vi "oax_gsTacho Analyzer.vi"() -> ()   [LabVIEW 2017]
doc: "<B>Tach Signal Analyzer</B>\n\nUse the Tach Signal Analyzer to prepare data samples for order tracking. The raw data can be input from either a binary NI-DAQ file collected by the <B>DSA Data Logger</B> or a general Windows .wav file. In this demo application, the usable data is limited to the data files come along with it.\n\nBy adjusting the <B>Selected Order</B> control in the <B>Time-Frequency Plot Parameters</B> section of the front panel, you can see a black curve moving around in the <B>Time-Frequency Plot</B>. The black curve represents the instantaneous frequencies of the selected order. You can increase the mask width to make the black curve more visible. For accurate order tracking, the black curve must be right on top of the corresponding orders displayed in the <B>Time-Frequency Plot</B>. You can use the controls in the <B>Tachometer Control</B> section to alter the black curve for a better fit.\n\nIn addition to verifying computed instantaneous frequencies, the <B>Tach Signal Analyzer</B> also allows you to select the most interesting events and to remove unwanted samples from the data record. For the sake of computation speed, it is important to keep the number of analyzed data samples as small as possible.\n\nOnce you have a good fit of the black curve on the corresponding orders in the <B>Time-Frequency Plot</B>, choose <B>File >> Save</B> on the toolbar to create an intermediate data file for order analysis."
uses:
  <vilib>/addons/Sound and Vibration/Order Analysis/Tach Process/SubVIs/speed profile.ctl
  <vilib>/addons/Sound and Vibration/Order Analysis/Ref Gabor Order Tracking/window information.ctl
  <vilib>/Analysis/1siggen.llb/Ramp Pattern by Samples.vi
  <vilib>/addons/Sound and Vibration/Order Analysis/Ref Gabor Order Tracking/Get Freq-Time Spectral Map (U8).vi
  Instance           2 28Saved   oax_gsTacho Analyzer .vi
  Instance           1 28Saved   oax_gsTacho Analyzer .vi
  <vilib>/addons/Sound and Vibration/Order Analysis/Example Support/Demo VI/Start-Up Kit/OAT Start/global variable.vi
  <vilib>/addons/Sound and Vibration/Order Analysis/Tach Process/SoundVib_TachProcess.lvlib
  <vilib>/addons/Sound and Vibration/Order Analysis/Gabor Order Tracking/SoundVib_Gabor.lvlib
  <vilib>/Analysis/NI_AALBase.lvlib
panel:
  in  "Save":bool
  in  "Select Data":string(tree)="UpAcc.wav"
  out "check sum":i16[](array[numeric])
  out "file names":string[](array[string])
  in  "unit":u16(ring) items=["Order", "Hz"]
  in  "Bandwidth":dbl(slide)=0.5 min=0.0 scale=0.0..1.0 scale format="%.2p"
  out "window information":T1={"window type"=3, "window length"=1} {"window type" items=["None"=0, "Hanning"=1, "Hamming"=2, "Blackman-Harris"=3, "Exact Blackman"=4, "Blackman"=5, "Flat Top"=6, "4 Term B-Harris"=7, "7 Term B-Harris"=8, "Low Sidelobe"=9, "Gaussian"=62]; "window length" min=0}
  out "Sample Rate (Hz)":dbl
  out "S&V plot":dbl[](graph)
  in  "Missing\nPulses?":bool
  in  "Threshold":bool
  in  "threshold lvl":dbl
  out "Num. of Data Selected":i32
  out "file start":i32=414
  out "Status":string="Waiting ..."
  out "Pulse Info":T2 {"speed [RPM]" format="%.2f"; "time [s]" format="%.2f"}
  in  "Pulses/Rev":i32=2
  in  "Window Length":T3(ring)=enum."2048"
  in  "Selected Order":dbl=1.0 min=0.1 step=0.1 format="%.1f"
  in  "Slope":enum16{"Rise", "Fall"}(ring)
  in  "Detrend":dbl(slide) min=0.0 max=1.0 step=0.05 scale=0.0..1.0 scale format="%.2f"
  out "Sound or Vibration Data":string
  out "Tachometer Data":string
  out "tach plot":cluster{dbl[], dbl[]}[](graph)
  out "Time-Frequency Plot":u8[][](graph)
  # "Time-Frequency Plot \nParameters"
  # "narrow"
  # "wide"
  # "Tachometer Control"
  # "Save Data"
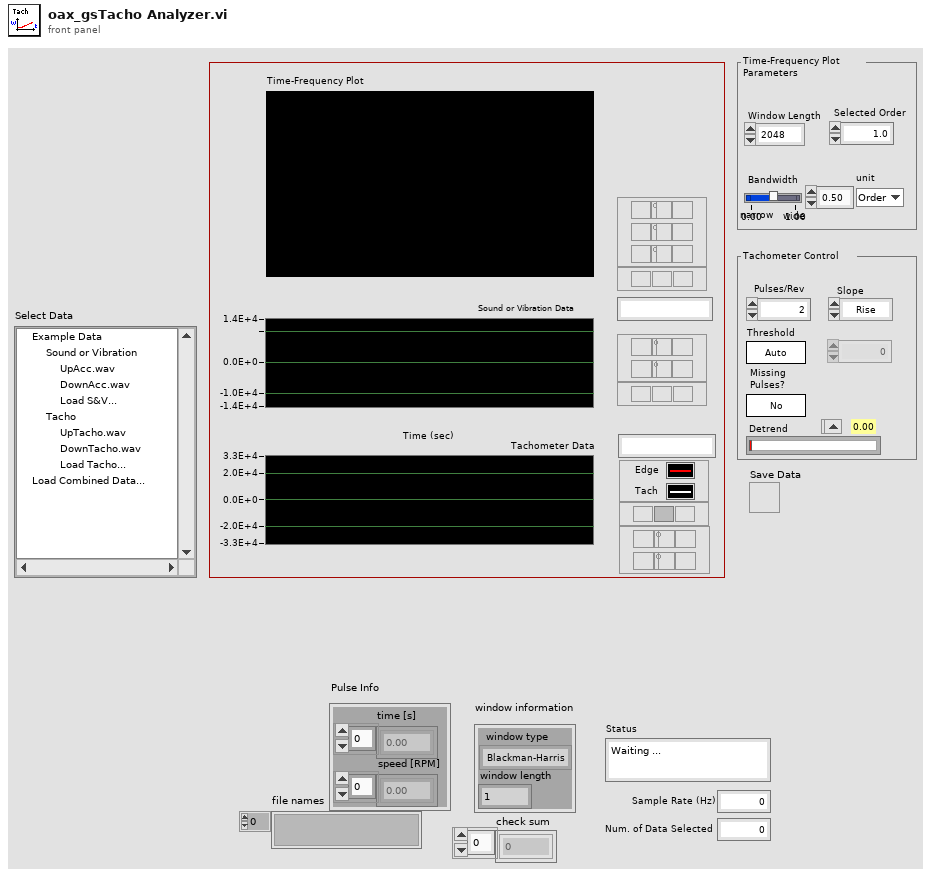
[diagram p1: front panel]
types:
  T1 = typedef "SoundVib_Gabor.lvlib/window information.ctl" = cluster{"window type":u32, "window length":i32}
  T2 = typedef "SoundVib_TachProcess.lvlib/speed profile.ctl" = cluster{"time [s]":dbl[], "speed [RPM]":dbl[]}
  T3 = enum16{"1024", "2048", "4096", "8192", "16384", "32768"}
  T4 = cluster{"Tach processed":bool, "SV processed":bool, "sample rate":u32}
  T5 = cluster{"Bandwidth":dbl, "unit":u16, "Selected Order":dbl}
  T6 = cluster{"Pulses/Rev":i32, "Detrend":dbl, "Slope":enum16{"Rise", "Fall"}, "Missing\nPulses?":bool, "threshold lvl":dbl, "Threshold":bool}
  T7 = typedef "Sound Format+.ctl" = cluster{"quality":enum16{"mono", "stereo"}, "sample rate":u32, "bits/sample":enum16{"8 bit", "16 bit"}}
  T8 = typedef "SoundVib_Gabor.lvlib/GT RefNum.ctl" = refnum<k1>
  T9 = cluster{"name":string, "multiplier":sgl, "offset":sgl, "sensor sensitivity (mV/EU)":dbl, "engineering units":enum16{"custom...", "V", "Pa", "g", "m/s^2", "m/s", "m", "in/s^2", "in/s", "in"}}[]
  T10 = cluster{"YScale.NameLbl.Text":string, "YScale.NameLbl.Text":string}
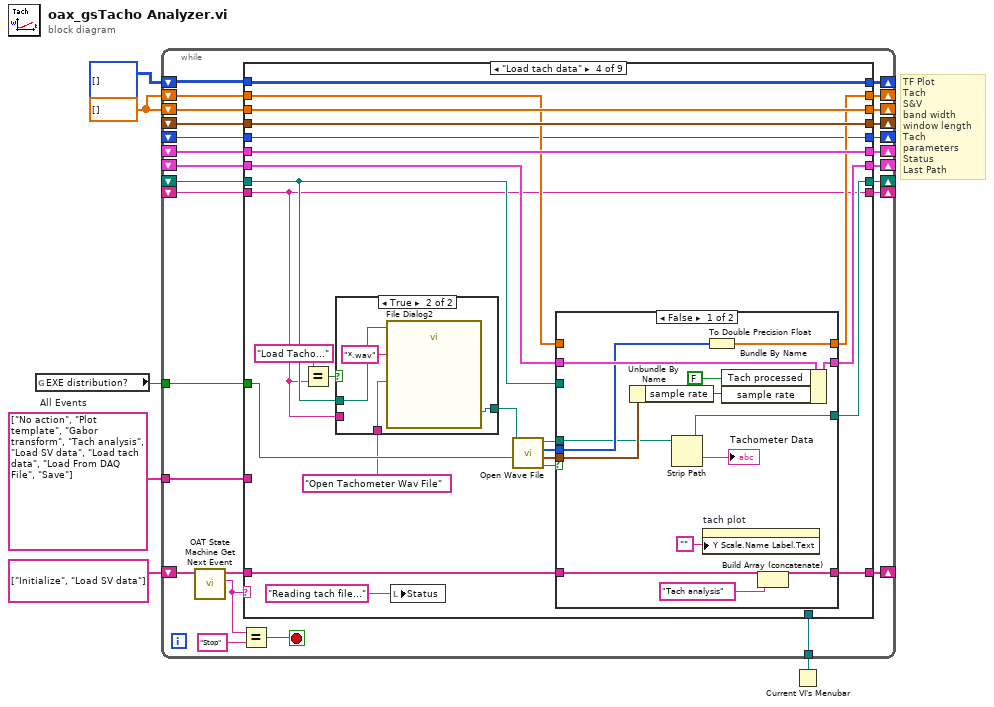
[diagram p0: block diagram]
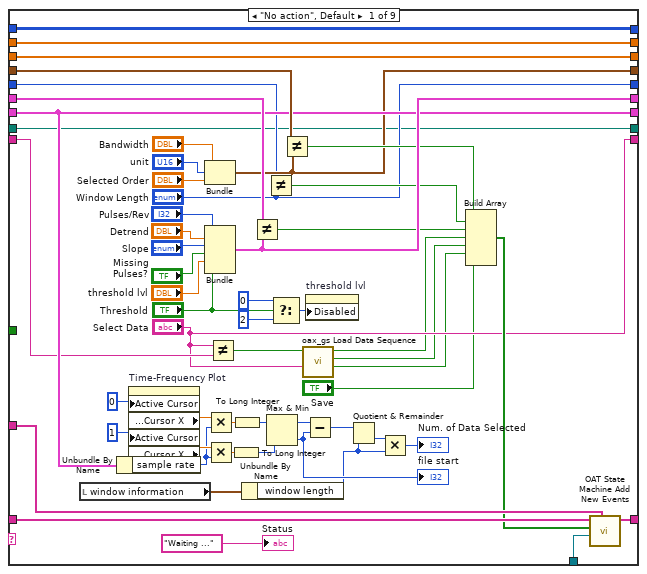
[diagram p2: hidden frame]
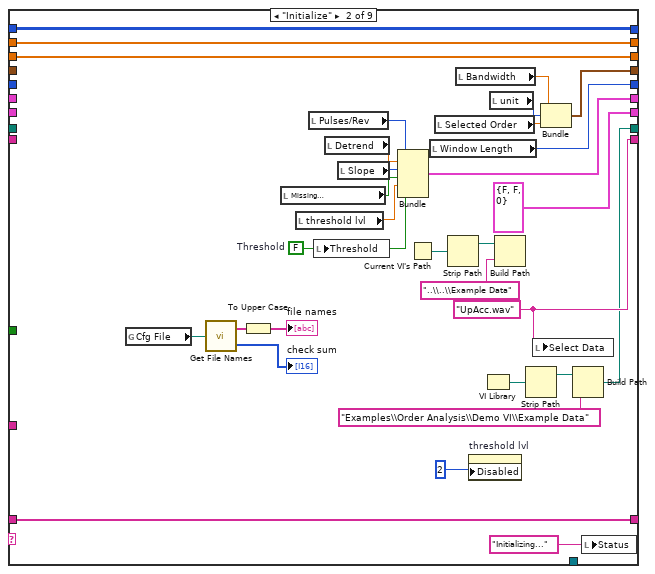
[diagram p3: hidden frame]
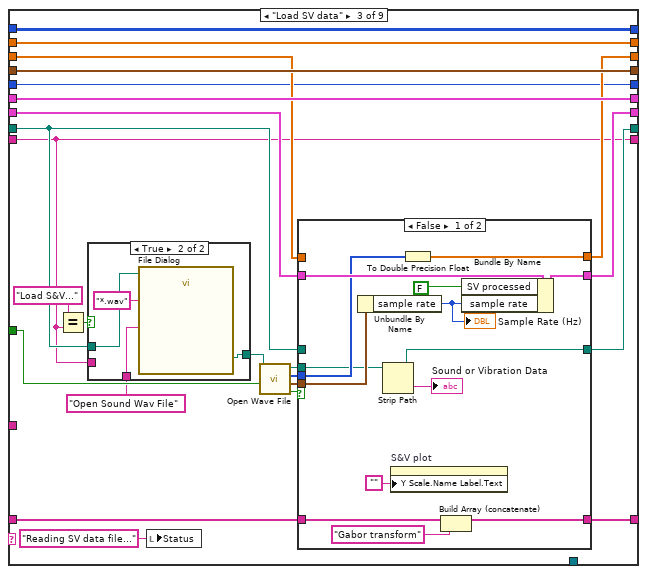
[diagram p4: hidden frame]
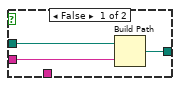
[diagram p5: hidden frame]
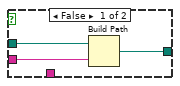
[diagram p7: hidden frame]
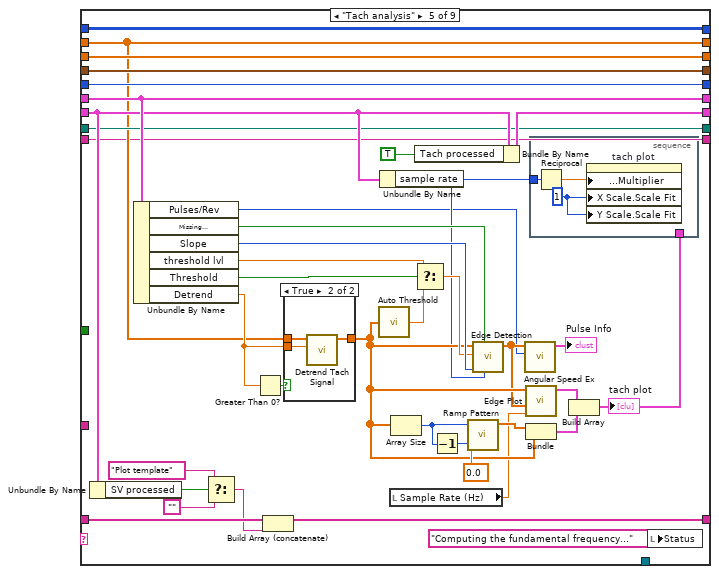
[diagram p9: hidden frame]
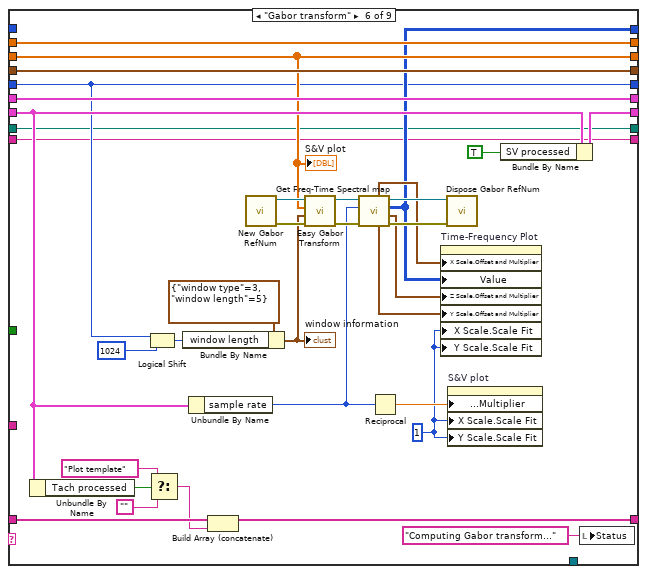
[diagram p11: hidden frame]
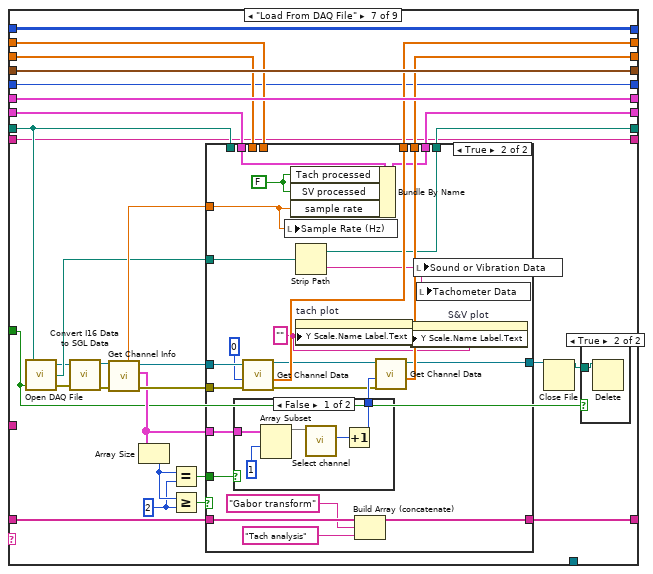
[diagram p12: hidden frame]
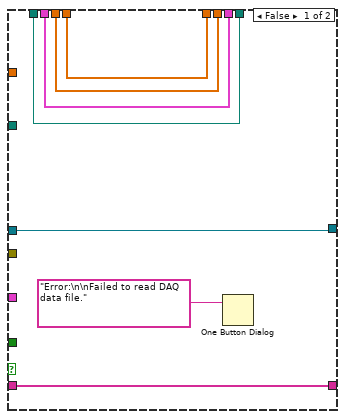
[diagram p14: hidden frame]
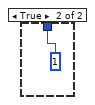
[diagram p15: hidden frame]
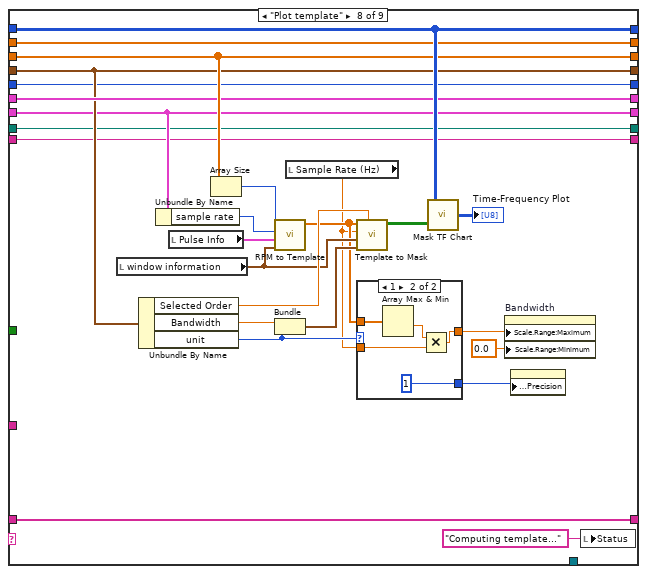
[diagram p16: hidden frame]
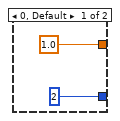
[diagram p17: hidden frame]
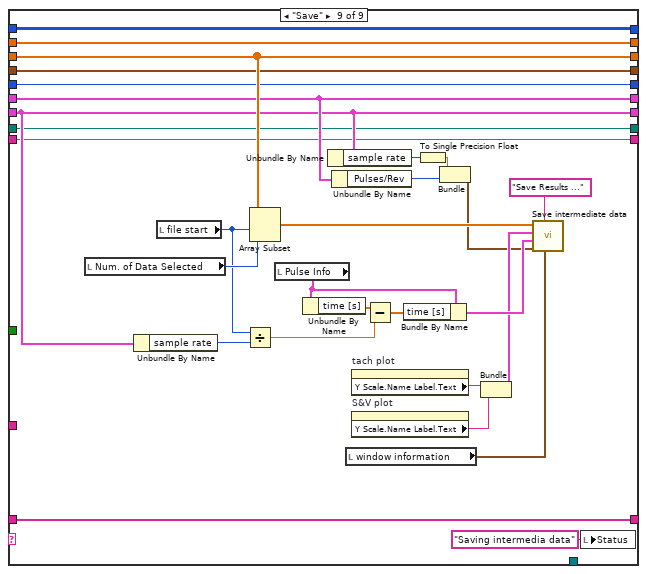
[diagram p18: hidden frame]
diagram:
  w5 = dbl[] [] ("data")
  w4 = string[] ["No action", "Plot template", "Gabor transform", "Tach analysis", "Load SV data", "Load tach data", "Load From DAQ File", "Save"]  # All Events
  # "TF Plot\nTach\nS&V\nband width\nwindow length\nTach parameters\nStatus\nLast Path"
  n1 = global read "global variable.vi" "EXE distribution?"() -> (w1:bool)
  n2 = Current VI's Menubar() -> (w2:refnum<k9>)
  n3 = while {
    tunnel: w1 -> [w9]
    shift-left: _ -> [w11]
    shift-right: [w10] -> _
    shift-left: _ -> [w12]
    shift-right: [w13] -> _
    shift-left: _ -> [w14]
    shift-right: [w16] -> _
    tunnel: w2 -> [w17]
    shift-left: _ -> [w18]
    shift-right: [w21] -> _
    shift-left: _ -> [w19]
    shift-right: [w20] -> _
    tunnel: w4 -> [w27]
    shift-left: string[] ["Initialize", "Load SV data"] ("Event Queue Out") -> [w28]
    shift-right: [w25] -> _
    shift-left: w5 -> [w15]
    shift-right: [w29] -> _
    shift-left: w5 -> [w30]
    shift-right: [w31] -> _
    shift-left: u8[][] [] ("graph [U8]") -> [w32]
    shift-right: [w33] -> _
    shift-right: [w8] -> _
    shift-left: _ -> [w7]
    stop <- w23 stop-if-true
    n4 = call <vilib>:"OAT State Machine Get Next Event.vi"("event queue in"=w28) -> ("next event"=w24:string, "event queue out"=w26:string[])  [unwired: 5 in]
    n5 = Equal?(x=w24, y="Stop" ("item tag")) -> (x = y?=w23:bool)
    n6 = case shown="\"Load tach data\"" w24 {
      tunnel: [w88 w118 w143 w192 w256 w274 w328 w389 w427] -> w33
      tunnel: w32 -> [w88 w118 w143 w192 w256 _ w328 w389 w427]
      tunnel: [w87 w117 w142 w187 w222 w292 w323 w387 w426] -> w31
      tunnel: w30 -> [w87 w117 w142 w184 w222 w292 w318 w387 w426]
      tunnel: [w86 w116 w135 w191 w247 w279 w316 w386 w425] -> w29
      tunnel: w27 -> [w85 _ _ _ _ _ _ _ _]
      tunnel: w26 -> [w84 w115 w141 w186 w246 w290 w322 w385 w419]
      tunnel: [w83 w115 w140 w185 w245 w289 w313 w385 w419] -> w25
      tunnel: [w81 w105 w137 w188 w237 w287 w326 w382 w414] -> w21
      tunnel: [w47 w107 w138 w189 w238 w286 w327 w381 w415] -> w20
      tunnel: w19 -> [w80 _ w138 w189 w238 w286 w327 w381 w415]
      tunnel: w18 -> [w79 _ w137 w188 w237 w287 w326 w382 w414]
      tunnel: w17 -> [w77 _ _ _ _ _ _ _ _]
      tunnel: w14 -> [w52 _ w133 w183 w227 w280 w310 w379 w413]
      tunnel: [w52 T4 {"Tach processed"=FALSE, "SV processed"=FALSE, "sample rate"=0} w132 w182 w228 w281 w311 w379 w413] -> w16
      tunnel: w15 -> [w86 w116 w134 w191 w247 w279 w315 w386 w425]
      tunnel: ["Window Length" w101 w131 w181 w224 w268 w308 w370 w401] -> w13
      tunnel: w12 -> [w46 _ w131 w181 w224 w268 w308 w370 w401]
      tunnel: w11 -> [w41 _ w124 w171 w223 w266 w307 w367 w400]
      tunnel: [w41 w89 w130 w180 w223 w266 w306 w367 w400] -> w10
      tunnel: w9 -> [_ _ w129 w178 _ _ w303 _ _]
      tunnel: ["Select Data" w93 w121 w170 w221 w264 w298 w366 w399] -> w8
      tunnel: w7 -> [w40 _ w121 w170 w221 w264 w298 w366 w399]
      frame "No action", Default {
        n7 = local read "window information"() -> (w43:T1)
        n8 = Unbundle By Name(w52) -> ("sample rate"=w51:u32)
        n9 = property on="Time-Frequency Plot" class="IntGraph (strict)"("Active Cursor"=u32 0 ("Write Attribute"), "Active Cursor"=u32 1 ("Write Attribute")) -> ("Cursor.Cursor Position:Cursor X"=w62:dbl, "Cursor.Cursor Position:Cursor X"=w61:dbl)  [unwired: 2 in, 2 out]
        n10 = Bundle("Bandwidth"="Bandwidth", "unit"="unit", "Selected Order"="Selected Order") -> (w47:T5)  [unwired: 1 in]
        n11 = Bundle("Pulses/Rev"="Pulses/Rev", "Detrend"="Detrend", "Slope"="Slope", "Missing\nPulses?"="Missing\nPulses?", "threshold lvl"="threshold lvl", "Threshold"="Threshold") -> (w81:T6)  [unwired: 1 in]
        n12 = Multiply(x=w62, y=w51) -> (x*y=w59:dbl)
        n13 = Multiply(x=w61, y=w51) -> (x*y=w60:dbl)
        n14 = Not Equal?(x="Select Data", y=w40) -> (x != y?=w39:bool)
        n15 = To Long Integer(number=w60) -> (32bit integer=w54:i32)
        n16 = To Long Integer(number=w59) -> (32bit integer=w55:i32)
        n17 = Unbundle By Name(w43) -> ("window length"=w42:i32)
        n18 = Not Equal?(x=w79, y=w81) -> (x != y?=w66:bool)
        n19 = Not Equal?(x=w46, y="Window Length") -> (x != y?=w45:bool)
        n20 = Max & Min(x=w55, y=w54) -> (max(x,y)=w56:i32, min(x,y)=w53:i32)
        "file start" <- w53
        n21 = Select(t=u8 0, s="Threshold", f=u8 2) -> (s? t:f=w74:u8)
        n22 = Not Equal?(x=w80, y=w47) -> (x != y?=w48:bool)
        n23 = call <vilib>:"oax_gs Load Data Sequence.vi"("Select Data"="Select Data", "value change"=w39) -> ("load from daq file"=w35:bool, "load tacho data"=w36:bool, "load sv data"=w37:bool)  [unwired: 7 in]
        n24 = Subtract(x=w56, y=w53) -> (x-y=w65:i32)
        n25 = property on="threshold lvl" class="DigNum (strict)"("Disabled"=w74) -> ()  [unwired: 2 in, 2 out]
        n26 = Quotient & Remainder(x=w65, y=w42) -> (floor(x/y)=w63:i32)  [unwired: 1 out]
        n27 = Multiply(x=w63, y=w42) -> (x*y=→"Num. of Data Selected":i32)
        n28 = Build Array(w48, w45, w66, w37, w36, w35, "Save") -> (w78:bool[])
        n29 = call <vilib>:"OAT State Machine Add New Events.vi"("Event Names"=w85, "Menu Refnum"=w77, "New Events"=w78, "Event Queue In"=w84) -> ("Event Queue Out"=w83:string[])  [unwired: 7 in]
        "Status" <- "Waiting ..."
      }
      frame "Initialize" {
        w93 = "UpAcc.wav" ("Select Data")
        w106 = FALSE  # Threshold
        n30 = global read "global variable.vi" "Cfg File"() -> (w97:path)
        n31 = call <vilib>:"Get File Names.vi"("configuration file path"=w97) -> ("file names"=w96:string[], "check sum"=→"check sum":i16[])
        n32 = To Upper Case(1:w96) -> (0:→"file names":string[])
        n33 = local read "Missing\nPulses?"() -> (w109:bool)
        n34 = local read "threshold lvl"() -> (w108:dbl)
        n35 = local read "Pulses/Rev"() -> (w112:i32)
        n36 = local write "Threshold"(w106) -> ()
        n37 = local read "Detrend"() -> (w111:dbl)
        n38 = local read "Slope"() -> (w110:enum16{"Rise", "Fall"})
        n39 = Bundle("Pulses/Rev"=w112, "Detrend"=w111, "Slope"=w110, "Missing\nPulses?"=w109, "threshold lvl"=w108, "Threshold"=w106) -> (w105:T6)  [unwired: 1 in]
        n40 = Current VI's Path() -> (path=w98:path)
        n41 = local read "Window Length"() -> (w101:T3)
        n42 = local read "Selected Order"() -> (w113:dbl)
        n43 = Strip Path(path=w98) -> (stripped path=w99:path)  [unwired: 1 out]
        n44 = local read "Bandwidth"() -> (w103:dbl)
        n45 = property on="threshold lvl" class="DigNum (strict)"("Disabled"=u8 2) -> ()  [unwired: 2 in, 2 out]
        n46 = VI Library() -> (path=w92:path)
        n47 = local read "unit"() -> (w102:u16)
        n48 = Build Path(base path=w99, name or relative path="..\\..\\Example Data") -> ()  [unwired: 1 out]
        n49 = Strip Path(path=w92) -> (stripped path=w91:path)  [unwired: 1 out]
        n50 = local write "Select Data"(w93) -> ()
        n51 = Bundle("Bandwidth"=w103, "unit"=w102, "Selected Order"=w113) -> (w107:T5)  [unwired: 1 in]
        n52 = Build Path(base path=w91, name or relative path="Examples\\Order Analysis\\Demo VI\\Example Data") -> (appended path=w89:path)
        n53 = local write "Status"("Initializing...") -> ()
      }
      frame "Load SV data" {
        n54 = Equal?(x="Load S&V...", y=w121) -> (x = y?=w122:bool)
        n55 = case shown="True" w122 {
          tunnel: [w144 w150] -> w125
          tunnel: w124 -> [w146 w148]
          tunnel: w121 -> [w145 _]
          tunnel: "Open Sound Wav File" ("prompt") -> [_ w147]
          frame False {
            n56 = Build Path(base path=w146, name or relative path=w145) -> (appended path=w144:path)
          }
          frame True {
            n57 = call "File Dialog"("start path"=w148, "prompt"=w147, "pattern (all files)"="*.wav") -> ("selected path"=w150:path)  [unwired: 9 in, 3 out]
          }
        }
        n58 = local write "Status"("Reading SV data file..." ("status")) -> ()
        n59 = call <vilib>:"Open Wave File.vi"("open original files"=w129, "start path"=w125) -> ("cancelled"=w128:bool, "sound format"=w126:T7, "wave data"=w127:i16[], "wave file path out"=w136:path)  [unwired: 6 in]
        n60 = case shown="False" w128 {
          tunnel: w141 -> [w164 w167]
          tunnel: [w162 w167] -> w140
          tunnel: w136 -> [w151 _]
          tunnel: [w161 w168] -> w135
          tunnel: w134 -> [_ w168]
          tunnel: w133 -> [w160 w166]
          tunnel: [w159 w166] -> w132
          tunnel: [w154 w165] -> w130
          tunnel: w124 -> [_ w165]
          tunnel: w127 -> [w153 _]
          tunnel: w126 -> [w152 _]
          frame False {
            n61 = Unbundle By Name(w152) -> ("sample rate"=w155:u32)
            "Sample Rate (Hz)" <- w155
            n62 = Strip Path(path=w151) -> (stripped path=w154:path, name=→"Sound or Vibration Data":string)
            n63 = property on="S&V plot" class="WFGraph (strict)"("Y Scale.Name Label.Text"="") -> ()  [unwired: 2 in, 2 out]
            n64 = To Double Precision Float(number=w153) -> (double precision float=w161:dbl[])
            n65 = Build Array (concatenate)(w164, "Gabor transform" ("status")) -> (w162:string[])
            n66 = Bundle By Name(cluster=w160, "SV processed"=FALSE, "sample rate"=w155) -> (w159:T4)
          }
          frame True {
          }
        }
      }
      frame "Load tach data" {
        n67 = Equal?(x="Load Tacho...", y=w170) -> (x = y?=w173:bool)
        n68 = case shown="True" w173 {
          tunnel: [w193 w199] -> w172
          tunnel: w171 -> [w195 w197]
          tunnel: w170 -> [w194 _]
          tunnel: "Open Tachometer Wav File" ("prompt") -> [_ w196]
          frame False {
            n69 = Build Path(base path=w195, name or relative path=w194) -> (appended path=w193:path)
          }
          frame True {
            n70 = call "File Dialog2"("start path"=w197, "prompt"=w196, "pattern (all files)"="*.wav") -> ("selected path"=w199:path)  [unwired: 9 in, 3 out]
          }
        }
        n71 = local write "Status"("Reading tach file..." ("status")) -> ()
        n72 = call <vilib>:"Open Wave File.vi"("open original files"=w178, "start path"=w172) -> ("cancelled"=w177:bool, "sound format"=w175:T7, "wave data"=w176:i16[], "wave file path out"=w179:path)  [unwired: 6 in]
        n73 = case shown="False" w177 {
          tunnel: [w204 w217] -> w187
          tunnel: w186 -> [w212 w216]
          tunnel: [w211 w216] -> w185
          tunnel: w184 -> [_ w217]
          tunnel: [w209 w215] -> w182
          tunnel: w183 -> [w210 w215]
          tunnel: w171 -> [_ w214]
          tunnel: [w205 w214] -> w180
          tunnel: w179 -> [w200 _]
          tunnel: w176 -> [w202 _]
          tunnel: w175 -> [w201 _]
          frame False {
            n74 = Unbundle By Name(w201) -> ("sample rate"=w203:u32)
            n75 = Strip Path(path=w200) -> (stripped path=w205:path, name=→"Tachometer Data":string)
            n76 = property on="tach plot" class="XYGraph (strict)"("Y Scale.Name Label.Text"="") -> ()  [unwired: 2 in, 2 out]
            n77 = To Double Precision Float(number=w202) -> (double precision float=w204:dbl[])
            n78 = Bundle By Name(cluster=w210, "Tach processed"=FALSE, "sample rate"=w203) -> (w209:T4)
            n79 = Build Array (concatenate)(w212, "Tach analysis" ("status")) -> (w211:string[])
          }
          frame True {
          }
        }
      }
      frame "Tach analysis" {
        n80 = Unbundle By Name(w227) -> ("SV processed"=w229:bool)
        n81 = Unbundle By Name(w237) -> ("Pulses/Rev"=w219:i32, "Missing\nPulses?"=w242:bool, "Slope"=w243:enum16{"Rise", "Fall"}, "threshold lvl"=w236:dbl, "Threshold"=w235:bool, "Detrend"=w239:dbl)
        n82 = Select(t="Plot template" ("status"), s=w229, f="") -> (s? t:f=w230:string)
        n83 = Greater Than 0?(x=w239) -> (x > 0?=w250:bool)
        n84 = Build Array (concatenate)(w246, w230) -> (w245:string[])
        n85 = case shown="True" w250 {
          tunnel: [w260 w263] -> w240
          tunnel: w222 -> [w260 w262]
          tunnel: w239 -> [_ w261]
          frame False {
          }
          frame True {
            n86 = call <vilib>:"Detrend Tach Signal.vi"("detrend level (0.0)"=w261, "x[n]"=w262) -> ("detrend"=w263:dbl[])  [unwired: 7 in, 2 out]
          }
        }
        n87 = call <vilib>:"Auto Threshold.vi"("x[n]"=w240) -> ("threshold"=w234:dbl)
        n88 = Unbundle By Name(w227) -> ("sample rate"=w226:u32)
        n89 = local read "Sample Rate (Hz)"() -> (w225:dbl)
        n90 = Array Size(array=w240) -> (size(s)=w255:i32)
        n91 = Bundle By Name(cluster=w227, "Tach processed"=TRUE ("Tach loaded")) -> (w228:T4)
        n92 = Select(t=w236, s=w235, f=w234) -> (s? t:f=w241:dbl)
        n93 = Decrement(x=w255) -> (x-1=w254:i32)
        n94 = call-poly <vilib>:"Ramp Pattern.vi"("start"=0.0, "end"=w254, "samples"=w255) -> ("Ramp Pattern"=w249:dbl[])  [unwired: 7 in, 1 out]
        n95 = call <vilib>:"Edge Detection.vi"("sampling frequency [Hz]"=w226, "missing pulses? (no:F)"=w242, "slope (Rise)"=w243, "threshold (0.0)"=w241, "x[n]"=w240) -> ("pulse positions [s]"=w220:dbl[])  [unwired: 5 in, 1 out]
        n96 = call <vilib>:"Angular Speed Ex.vi"("pulse/revolution (1)"=w219, "pulse positions [s]"=w220) -> ("speed profile"=→"Pulse Info":T2)  [unwired: 8 in, 1 out]
        n97 = call <vilib>:"Edge Plot.vi"("sample rate [Hz]"=w225, "time instant\nof pulses"=w220, "Tach signal"=w240) -> ("Edge Plot"=w248:cluster{"X":dbl[], "Y":dbl[]})  [unwired: 4 in]
        n98 = Bundle("Ramp Pattern"=w249, "detrend"=w240) -> (w252:cluster{"Ramp Pattern":dbl[], "detrend":dbl[]})  [unwired: 1 in]
        n99 = Build Array(w248, w252) -> (w251:cluster{"Ramp Pattern":dbl[], "detrend":dbl[]}[])
        "tach plot" <- w251
        n100 = stacked-sequence {
          tunnel: w226 -> [w258]
          tunnel: w251 -> [_]
          frame #0 {
            w257 = u8 1 ("X Scale.Scale Fit")
            n101 = Reciprocal(x=w258) -> (1/x=w259:dbl)
            n102 = property on="tach plot" class="XYGraph (strict)"("X Scale.Offset and Multiplier:Multiplier"=w259, "X Scale.Scale Fit"=w257, "Y Scale.Scale Fit"=w257) -> ()  [unwired: 2 in, 2 out]
          }
        }
        n103 = local write "Status"("Computing the fundamental frequency..." ("status")) -> ()
      }
      frame "Gabor transform" {
        w265 = u8 1 ("X Scale.Scale Fit")
        n104 = Unbundle By Name(w280) -> ("Tach processed"=w277:bool)
        n105 = Logical Shift(y=w268, x=1024) -> (x << y=w269:i32)
        n106 = Select(t="Plot template" ("status"), s=w277, f="") -> (s? t:f=w283:string)
        n107 = Bundle By Name(cluster=T1 {"window type"=3, "window length"=5} ("window information"), "window length"=w269) -> (w270:T1)
        "window information" <- w270
        n108 = Unbundle By Name(w280) -> ("sample rate"=w276:u32)
        n109 = Build Array (concatenate)(w290, w283) -> (w289:string[])
        n110 = call <vilib>:"New Gabor RefNum.vi"() -> ("error out"=w293:errorcluster, "RefNum"=w297:T8)  [unwired: 9 in]
        n111 = call <vilib>:"Easy Gabor Transform.vi"("error in (no error)"=w293, "window info"=w270, "x[n]"=w279, "RefNum in"=w297) -> ("error out"=w295:errorcluster, "RefNum out"=w294:T8)  [unwired: 3 in, 3 out]
        n112 = call-poly <vilib>:"Get Freq-Time Spectral map.vi"("error in (no error)"=w295, "sampling frequency [Hz]"=w276, "RefNum in"=w294) -> ("error out"=w291:errorcluster, "quantization info"=w273:cluster{"offset":dbl, "multiplier":dbl}, "spectral map"=w274:u8[][], "RefNum out"=w296:T8, "frequency scale"=w272:cluster{"offset":dbl, "multiplier":dbl}, "time scale"=w275:cluster{"offset":dbl, "multiplier":dbl})  [unwired: 3 in]
        n113 = Reciprocal(x=w276) -> (1/x=w278:dbl)
        n114 = property on="Time-Frequency Plot" class="IntGraph (strict)"("X Scale.Offset and Multiplier"=w275, "Value"=w274, "Z Scale.Offset and Multiplier"=w273, "Y Scale.Offset and Multiplier"=w272, "X Scale.Scale Fit"=w265, "Y Scale.Scale Fit"=w265) -> ()  [unwired: 2 in, 2 out]
        n115 = call <vilib>:"Dispose Gabor RefNum.vi"("error in (no error)"=w291, "RefNum in"=w296) -> ()  [unwired: 6 in, 1 out]
        n116 = property on="S&V plot" class="WFGraph (strict)"("X Scale.Offset and Multiplier:Multiplier"=w278, "X Scale.Scale Fit"=w265, "Y Scale.Scale Fit"=w265) -> ()  [unwired: 2 in, 2 out]
        n117 = Bundle By Name(cluster=w280, "SV processed"=TRUE ("SV loaded")) -> (w281:T4)
        n118 = local write "Status"("Computing Gabor transform..." ("status")) -> ()
        "S&V plot" <- w279
      }
      frame "Load From DAQ File" {
        w319 = 2 ("y")
        n119 = call <vilib>:"Open DAQ File.vi"("EXE distribution?"=w303, "start path"=w307) -> ("error out"=w301:errorcluster, "new file path"=w305:path, "refnum out"=w302:refnum<file>)  [unwired: 1 in]
        n120 = call <vilib>:"Convert I16 Data to SGL Data.vi"("error in"=w301, "refnum in"=w302) -> ("error out"=w300:errorcluster, "refnum out"=w299:refnum<file>)  [unwired: 4 in]
        n121 = call <vilib>:"Get Channel Info.vi"("error in"=w300, "refnum in"=w299) -> ("error out"=w324:errorcluster, "channel information"=w312:T9, "dup refnum"=w325:refnum<file>, "Sample rate"=w309:sgl)  [unwired: 4 in, 2 out]
        n122 = Array Size(array=w312) -> (size(s)=w320:i32)
        n123 = Equal?(x=w320, y=w319) -> (x = y?=w317:bool)
        n124 = Greater Or Equal?(x=w320, y=w319) -> (x >= y?=w321:bool)
        n125 = case shown="True" w321 {
          tunnel: w325 -> [w333 w359]
          tunnel: w324 -> [_ w358]
          tunnel: [w335 w356] -> w323
          tunnel: w322 -> [w334 w349]
          tunnel: w318 -> [w335 _]
          tunnel: w317 -> [_ w355]
          tunnel: [w336 w351] -> w316
          tunnel: w315 -> [w336 _]
          tunnel: [w333 w350] -> w314
          tunnel: [w334 w347] -> w313
          tunnel: w312 -> [_ w346]
          tunnel: [w332 w344] -> w311
          tunnel: w310 -> [w332 w343]
          tunnel: w309 -> [_ w341]
          tunnel: w307 -> [w330 _]
          tunnel: [w330 w339] -> w306
          tunnel: w305 -> [_ w338]
          frame False {
            n126 = One Button Dialog(message="Error:\n\nFailed to read DAQ data file.") -> ()  [unwired: 1 in, 1 out]
          }
          frame True {
            w337 = "" ("Y Scale.Name Label.Text")
            w342 = FALSE
            n127 = case shown="False" w355 {
              tunnel: [w360 1 ("index")] -> w354
              tunnel: w346 -> [w364 _]
              frame False {
                n128 = Array Subset(array=w364, index=1) -> (w362:T9)  [unwired: 1 in]
                n129 = call <vilib>:"Select channel.vi"("Channel Info"=w362) -> ("index"=w361:i32)  [unwired: 5 in, 1 out]
                n130 = Increment(x=w361) -> (x+1=w360:i32)
              }
              frame True {
              }
            }
            n131 = call <vilib>:"Get Channel Data.vi"("error in"=w358, "index"=0, "refnum in"=w359) -> ("error out"=w352:errorcluster, "data"=w356:dbl[], "refnum out"=w353:refnum<file>)  [unwired: 3 in, 3 out]
            n132 = local write "Sample Rate (Hz)"(w341) -> ()
            n133 = Bundle By Name(cluster=w343, "Tach processed"=w342, "SV processed"=w342, "sample rate"=w341) -> (w344:T4)
            n134 = Strip Path(path=w338) -> (stripped path=w339:path, name=w340:string)
            n135 = property on="tach plot" class="XYGraph (strict)"("Y Scale.Name Label.Text"=w337) -> ()  [unwired: 2 in, 2 out]
            n136 = Build Array (concatenate)(w349, "Gabor transform" ("status"), "Tach analysis" ("status")) -> (w347:string[])
            n137 = call <vilib>:"Get Channel Data.vi"("error in"=w352, "index"=w354, "refnum in"=w353) -> ("data"=w351:dbl[], "refnum out"=w350:refnum<file>)  [unwired: 3 in, 4 out]
            n138 = property on="S&V plot" class="WFGraph (strict)"("Y Scale.Name Label.Text"=w337) -> ()  [unwired: 2 in, 2 out]
            n139 = local write "Sound or Vibration Data"(w340) -> ()
            n140 = local write "Tachometer Data"(w340) -> ()
          }
        }
        n141 = Close File(refnum=w314) -> (path=w304:path)  [unwired: 1 in, 1 out]
        n142 = case shown="True" w303 {
          tunnel: w304 -> [_ w329]
          frame False {
          }
          frame True {
            n143 = Delete(path (use dialog)=w329) -> ()  [unwired: 4 in, 3 out]
          }
        }
      }
      frame "Plot template" {
        n144 = local read "window information"() -> (w377:T1)
        n145 = Unbundle By Name(w381) -> ("Selected Order"=w380:dbl, "Bandwidth"=w376:dbl, "unit"=w374:u16)
        n146 = Unbundle By Name(w379) -> ("sample rate"=w378:u32)
        n147 = local read "Pulse Info"() -> (w383:T2)
        n148 = Array Size(array=w386) -> (size(s)=w391:i32)
        n149 = call <vilib>:"RPM to Template.vi"("window info"=w377, "speed profile"=w383, "sampling frequency [Hz]"=w378, "signal length"=w391) -> ("Gabor template"=w373:dbl[])  [unwired: 6 in, 1 out]
        n150 = Bundle("Bandwidth"=w376, "unit"=w374) -> (w375:cluster{"Bandwidth":dbl, "unit":u16})  [unwired: 1 in]
        n151 = local read "Sample Rate (Hz)"() -> (w372:dbl)
        n152 = call <vilib>:"Template to Mask.vi"("order (1.0)"=w380, "bandwidth"=w375, "window info"=w377, "sampling frequency [S/s]"=w372, "Gabor template"=w373) -> ("mask array"=w390:bool[][])  [unwired: 6 in]
        n153 = case shown="1" w374 {
          tunnel: w373 -> [_ w398]
          tunnel: w372 -> [_ w396]
          tunnel: [1.0 w395] -> w371
          tunnel: [u8 2 u8 1] -> w369
          frame 0, Default {
          }
          frame 1 {
            n154 = Array Max & Min(array=w398) -> (min value=w397:dbl)  [unwired: 3 out]
            n155 = Multiply(x=w397, y=w396) -> (x*y=w395:dbl)
          }
        }
        n156 = call <vilib>:"Mask TF Chart.vi"("Mask Array"=w390, "TF plot"=w389) -> ("TF plot Out"=→"Time-Frequency Plot":u8[][])
        n157 = property on="Bandwidth" class="Slide (strict)"("Scale.Range:Maximum"=w371, "Scale.Range:Minimum"=0.0) -> ()  [unwired: 2 in, 2 out]
        n158 = property class="DigNum (strict)"("Format & Precision:Precision"=w369) -> ()  [unwired: 2 in, 2 out]
        n159 = local write "Status"("Computing template..." ("status")) -> ()
      }
      frame "Save" {
        n160 = local read "Num. of Data Selected"() -> (w423:i32)
        n161 = Unbundle By Name(w413) -> ("sample rate"=w412:u32)
        n162 = local read "file start"() -> (w418:i32)
        n163 = Divide(x=w418, y=w412) -> (x/y=w416:dbl)
        n164 = Array Subset(array=w425, index=w418, length=w423) -> (w424:dbl[])
        n165 = local read "Pulse Info"() -> (w420:T2)
        n166 = Unbundle By Name(w420) -> ("time [s]"=w422:dbl[])
        n167 = Unbundle By Name(w413) -> ("sample rate"=w411:u32)
        n168 = Unbundle By Name(w414) -> ("Pulses/Rev"=w410:i32)
        n169 = local read "window information"() -> (w402:T1)
        n170 = property on="tach plot" class="XYGraph (strict)"() -> ("Y Scale.Name Label.Text"=w407:string)  [unwired: 2 in, 2 out]
        n171 = property on="S&V plot" class="WFGraph (strict)"() -> ("Y Scale.Name Label.Text"=w406:string)  [unwired: 2 in, 2 out]
        n172 = Subtract(x=w422, y=w416) -> (x-y=w421:dbl[])
        n173 = Bundle By Name(cluster=w420, "time [s]"=w421) -> (w408:T2)
        n174 = To Single Precision Float(number=w411) -> (single precision float=w404:sgl)
        n175 = Bundle(w404, "Pulses/Rev"=w410) -> (w403:cluster{sgl, "Pulses/Rev":i32})  [unwired: 1 in]
        n176 = Bundle("YScale.NameLbl.Text"=w407, "YScale.NameLbl.Text"=w406) -> (w405:T10)  [unwired: 1 in]
        n177 = call <vilib>:"Save intermediate data.vi"("window info"=w402, "prompt"="Save Results ..." ("Prompt"), "parameters"=w403, "speed profile"=w408, "lables"=w405, "S&V samples"=w424) -> ()  [unwired: 5 in, 1 out]
        n178 = local write "Status"("Saving intermedia data" ("status")) -> ()
      }
    }
  }
